vi "Test Cases - Cluster Changed Value as Arguments.vi"() -> ()   [LabVIEW 2017]
uses:
  6aef6293-1b46-43cc-a090-3bd41170cef4.vi
  c2ea3052-9718-4095-9bf2-a156dcd4a46a.vi
  API-String-Arugments-Support/_Support/Data To API String Arguments.vi
  API-String-Arugments-Support/_Support/Convert API String Arguments to Data(variant).vi
panel:
  out "Data":T1
  in  "With Reference Cluster Data":bool
  in  "Generate":bool
  in  "Reference cluster data":T1={"Name"="abc", "Child"={"Name"="ddd"}, "Bool"=FALSE}
  out "String 16":string="Bool:Off;child.name:ddd"
  out "error 9":errorcluster
  in  "Data 8":T1={"Name"="abc", "Child"={"Name"="ddd"}, "Bool"=FALSE}
  # "===>>"
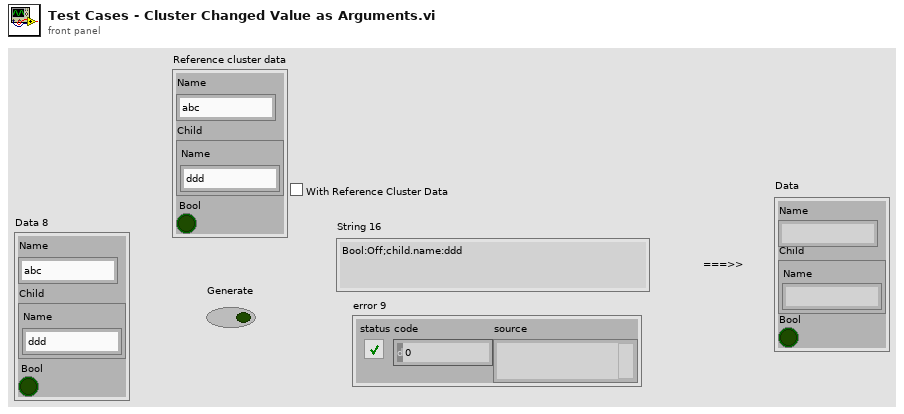
[diagram p1: front panel]
types:
  T1 = cluster{"Name":string, "Child":cluster{"Name":string}, "Bool":bool}
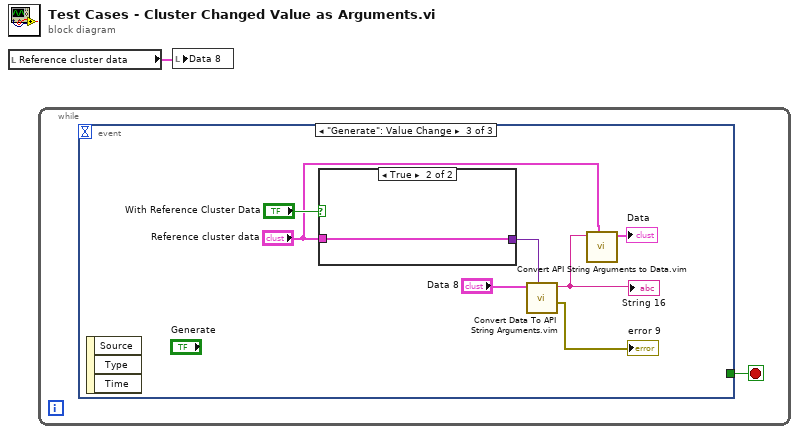
[diagram p0: block diagram]
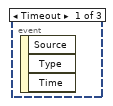
[diagram p2: hidden frame]
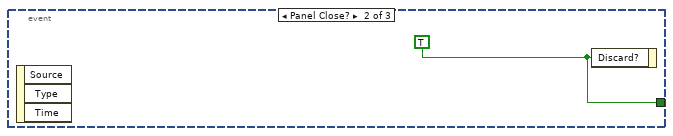
[diagram p3: hidden frame]
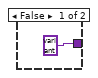
[diagram p4: hidden frame]
diagram:
  n1 = local read "Reference cluster data"() -> (w1:T1)
  n2 = while {
    stop <- w2 stop-if-true
    n3 = event shown="[2] \"Generate\": Value Change" {
      selector: _ -> [_ _ _]
      dyn-events: _ -> [_ _ _]
      timeout: _ -> [_ _ _]
      tunnel: [_ w3 _] -> w2
      event Timeout {
        n4 = event-data() -> ()  [unwired: 1 in, 3 out]
      }
      event Panel Close? {
        w3 = TRUE ("Discard?")
        n5 = event-data() -> ()  [unwired: 1 in, 3 out]
        n6 = event-data("Discard?"=w3) -> ()  [unwired: 1 in, 1 out]
      }
      event "Generate": Value Change {
        n7 = event-data() -> ()  [unwired: 1 in, 3 out]
        n8 = case shown="True" "With Reference Cluster Data" {
          tunnel: [variant w12] -> w7
          tunnel: "Reference cluster data" -> [_ w12]
          frame False {
          }
          frame True {
          }
        }
        n9 = call "Convert Data To API String Arguments.vim"("reference cluster data"=w7, "data"="Data 8") -> ("error out"=→"error 9":errorcluster, "String"=w6:string)  [unwired: 6 in]
        "String 16" <- w6
        n10 = call "Convert API String Arguments to Data.vim"("Type"="Reference cluster data", "String"=w6) -> ("Data"=→"Data":T1)  [unwired: 6 in, 1 out]
      }
    }
  }
  n11 = local write "Data 8"(w1) -> ()
